vi "Teleop.vi"(10 "Match Info":T1={"Autonomous Elapsed Seconds"=0.0, "TeleOp Elapsed Seconds"=0.0, "Disabled Elapsed Seconds"=0.0, "Visited Autonomous"=FALSE, "Visited TeleOp"=FALSE, "Visited Disabled"=FALSE, "Autonomous Settings"={"Autonomous Style"=enum."Independent", "VI Refnum"=refnum}}, 11 "Call Context":T2) -> ()   [LabVIEW 2011]
doc: "This VI is called for each TeleOp packet received from the DS where the robot is not disabled. It is often used to read from the joysticks and update I/O or to update setpoints for timed control loops. It should complete and return within 20 milliseconds or it may miss DS packets."
uses:
  <vilib>/Rock Robotics/WPI/DriverStation/WPI_DriverStationDerivedRobotMode.ctl
  <vilib>/Rock Robotics/WPI/DriverStation/WPI_DriverStationMatch Info.ctl
  Robot Global Data.vi
  System Set Points and States.vi
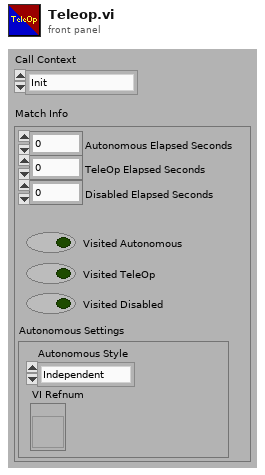
[diagram p1: front panel]
types:
  T1 = typedef "WPI_DriverStationMatch Info.ctl" = cluster{"Autonomous Elapsed Seconds":dbl, "TeleOp Elapsed Seconds":dbl, "Disabled Elapsed Seconds":dbl, "Visited Autonomous":bool, "Visited TeleOp":bool, "Visited Disabled":bool, "Autonomous Settings":cluster{"Autonomous Style":enum16{"Iterative", "Independent"}, "VI Refnum":refnum<vi>}}
  T2 = typedef "WPI_DriverStationDerivedRobotMode.ctl" = enum16{"Init", "Execute", "Stop"}
  T3 = typedef "WPI_JoystickDevRef.ctl" = cluster{"Device":T4}
  T4 = typedef "WPI_JoystickDeviceEnum.ctl" = enum16{"USB 1", "USB 2", "USB 3", "USB 4", "Kinect 1", "Kinect 2"}
  T5 = typedef "WPI_JoystickButtonState.ctl" = cluster{"Button 1":bool, "Button 2":bool, "Button 3":bool, "Button 4":bool, "Button 5":bool, "Button 6":bool, "Button 7":bool, "Button 8":bool, "Button 9":bool, "Button 10":bool, "Button 11":bool, "Button 12":bool}
  T6 = cluster{"axis 1 (x)":dbl, "axis 2 (y)":dbl, "axis 3 (throttle)":dbl, "axis 4":dbl, "axis 5":dbl, "axis 6":dbl}
  T7 = typedef "WPI_DigitalInputDevRef.ctl" = cluster{"DevStatus":errorcluster, "DIO Channel":T8, "Digital Module":T9}
  T8 = typedef "FPGA_DIOChannel.ctl" = enum8{"DIO 1", "DIO 2", "DIO 3", "DIO 4", "DIO 5", "DIO 6", "DIO 7", "DIO 8", "DIO 9", "DIO 10", "DIO 11", "DIO 12", "DIO 13", "DIO 14", "Invalid"}
  T9 = typedef "FPGA_TypedefDigitalModule.ctl" = enum16{"Digital Module 1", "Digital Module 2"}
  T10 = typedef "WPI_RobotDriveDevRef.ctl" = cluster{"DevStatus":errorcluster, "Motors[]":T11[], "Square Inputs":bool, "Max Output":dbl, "Isochronous":bool}
  T11 = typedef "WPI_MotorControlDeviceRef.ctl" = cluster{"DeviceStatus":errorcluster, "Type":enum16{"PWM", "CAN"}, "PWM":cluster{"Digital Module":T9, "PWM Channel":T12, "DeadBand":T13}, "CAN":cluster{"Device Number":u8, "Control Mode":T14, "Semaphore":T15, "Max Vout":dbl}, "Invert":bool, "TransformRef":T16, "InvTransformRef":T16}
  T12 = typedef "FPGA_DIOPWMChannel.ctl" = enum8{"PWM 1", "PWM 2", "PWM 3", "PWM 4", "PWM 5", "PWM 6", "PWM 7", "PWM 8", "PWM 9", "PWM 10", "Invalid"}
  T13 = typedef "WPI_PWMDeadband.ctl" = cluster{"Name":string, "maxPositivePwm":i32, "minPositivePwm":i32, "centerPwm":i32, "maxNegativePwm":i32, "minNegativePwm":i32, "angularRange":u16}
  T14 = typedef "WPI_CANJaguar_ControlMode.ctl" = enum8{"Percent VBus", "Current", "Speed", "Position", "Voltage"}
  T15 = typedef "Semaphore RefNum" = refnum<k1>
  T16 = typedef "WPI_PWMTransform_ConPane.ctl" = refnum<vi>
  T17 = cluster{"Position":cluster{"X":dbl, "Y":dbl}, "Distance (ft)":dbl}[]
  T18 = cluster{"Target Info[0]":cluster{"Position":cluster{"X":dbl, "Y":dbl}, "Distance (ft)":dbl}, "Target Info[1]":cluster{"Position":cluster{"X":dbl, "Y":dbl}, "Distance (ft)":dbl}, "Target Info[2]":cluster{"Position":cluster{"X":dbl, "Y":dbl}, "Distance (ft)":dbl}, "Target Info[3]":cluster{"Position":cluster{"X":dbl, "Y":dbl}, "Distance (ft)":dbl}, "Target Info[4]":cluster{"Position":cluster{"X":dbl, "Y":dbl}, "Distance (ft)":dbl}, "Target Info[5]":cluster{"Position":cluster{"X":dbl, "Y":dbl}, "Distance (ft)":dbl}, "Target Info[6]":cluster{"Position":cluster{"X":dbl, "Y":dbl}, "Distance (ft)":dbl}, "Target Info[7]":cluster{"Position":cluster{"X":dbl, "Y":dbl}, "Distance (ft)":dbl}, "Target Info[8]":cluster{"Position":cluster{"X":dbl, "Y":dbl}, "Distance (ft)":dbl}}
  T19 = typedef "WPI_AnalogChannelDevRef.ctl" = cluster{"DevStatus":errorcluster, "Analog Module":T20, "Analog Channel":T21}
  T20 = typedef "FPGA_TypedefAnalogModule.ctl" = enum16{"Analog Module 1", "Analog Module 2"}
  T21 = typedef "FPGA_AIChannel.ctl" = enum8{"AI 1", "AI 2", "AI 3", "AI 4", "AI 5", "AI 6", "AI 7", "AI 8", "Invalid"}
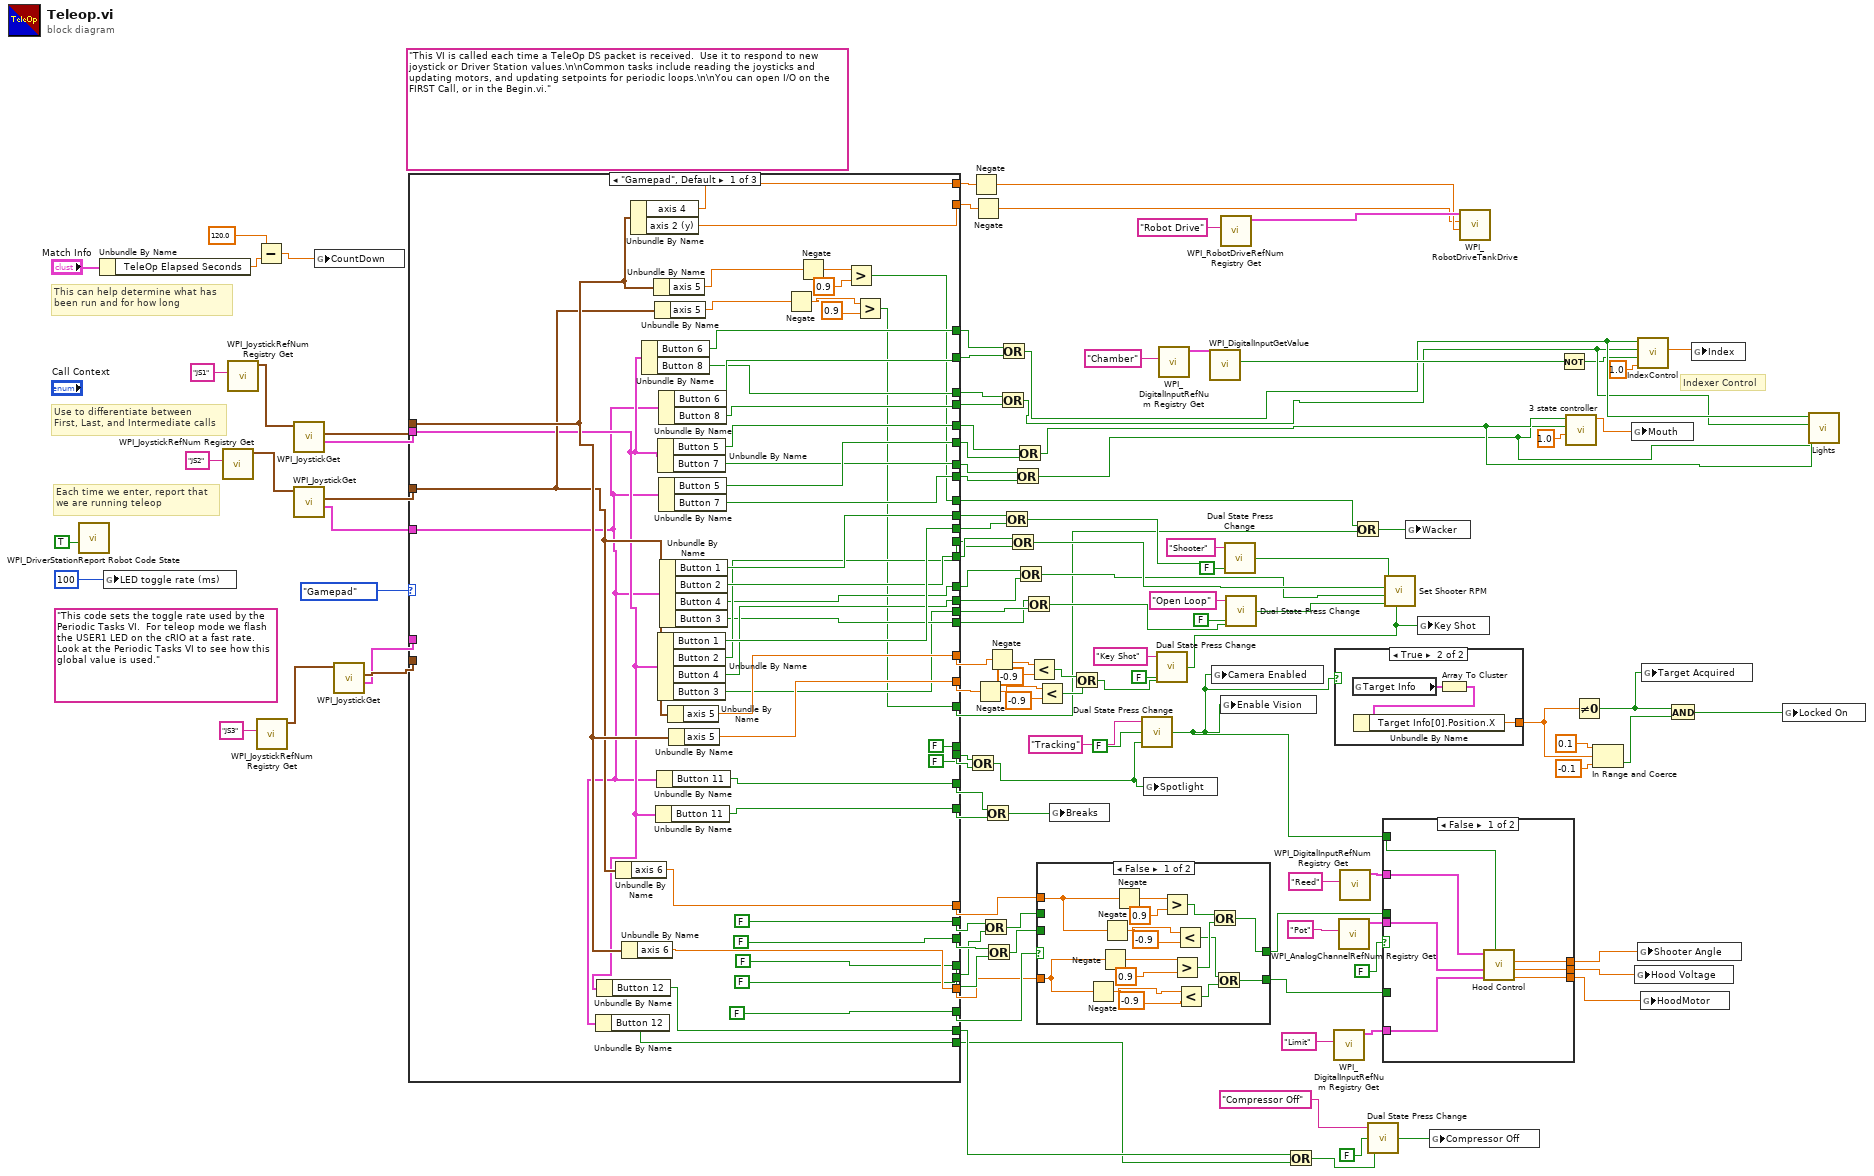
[diagram p0: block diagram]
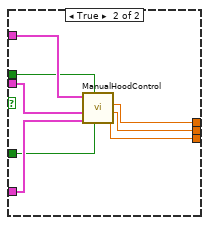
[diagram p2: hidden frame]
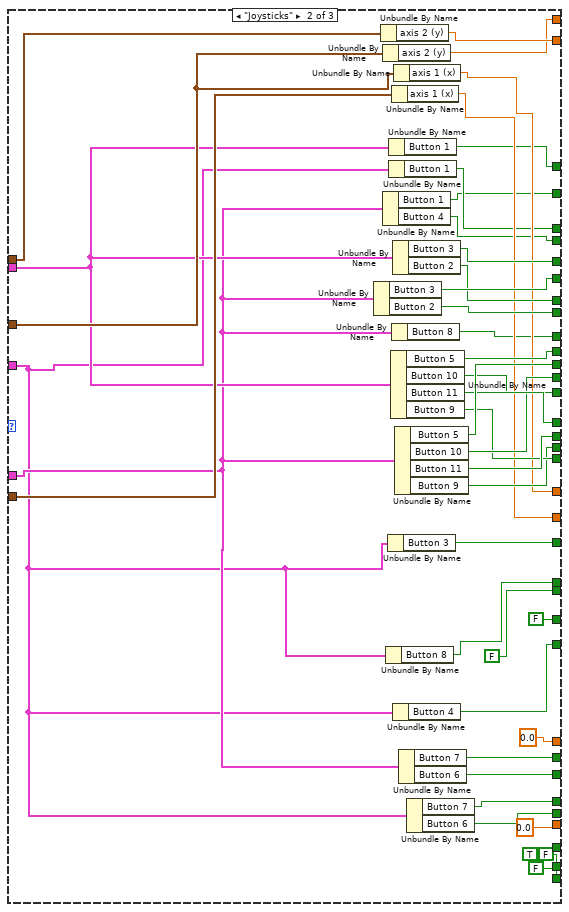
[diagram p4: hidden frame]
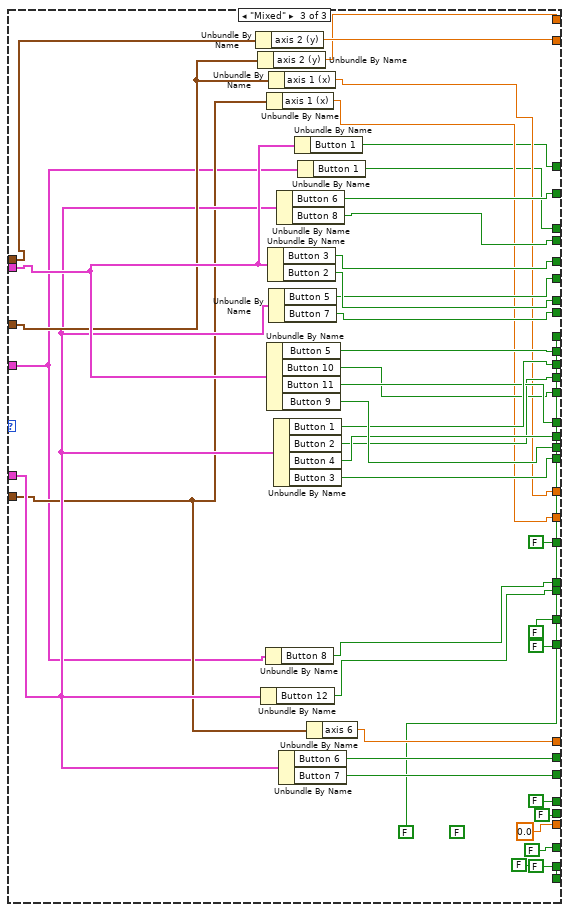
[diagram p5: hidden frame]
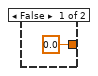
[diagram p6: hidden frame]
diagram:
  (unwired) "This code sets the toggle rate used by the Periodic Tasks VI.  For teleop mode we flash the USER1 LED on the cRIO at a fast rate.  Look at the Periodic Tasks VI to see how this global value is used."
  (unwired) "This VI is called each time a TeleOp DS packet is received.  Use it to respond to new joystick or Driver Station values.\n\nCommon tasks include reading the joysticks and updating motors, and updating setpoints for periodic loops.\n\nYou can open I/O on the FIRST Call, or in the Begin.vi."
  # "Indexer Control"
  # "Each time we enter, report that\nwe are running teleop"
  # "Use to differentiate between\nFirst, Last, and Intermediate calls"
  # "This can help determine what has\nbeen run and for how long"
  n1 = call <vilib>:"WPI_DriverStationReport Robot Code State.vi"("TeleOp"=TRUE ("Autonomous")) -> ()  [unwired: 10 in, 1 out]
  n2 = Unbundle By Name("Match Info") -> ("TeleOp Elapsed Seconds"=w95:dbl)
  n3 = global write "Robot Global Data.vi" "LED toggle rate (ms)"(u32 100 ("LED ms toggle rate")) -> ()
  n4 = call <vilib>:"WPI_JoystickRefNum Registry Get.vi"("refnum name"="JS2") -> ("JoystickDevRef"=w89:T3)  [unwired: 9 in, 1 out]
  n5 = call <vilib>:"WPI_JoystickRefNum Registry Get.vi"("refnum name"="JS1") -> ("JoystickDevRef"=w116:T3)  [unwired: 9 in, 1 out]
  n6 = Subtract(x=120.0, y=w95) -> (x-y=w61:dbl)
  n7 = call <vilib>:"WPI_JoystickRefNum Registry Get.vi"("refnum name"="JS3") -> ("JoystickDevRef"=w57:T3)  [unwired: 9 in, 1 out]
  n8 = call <vilib>:"WPI_JoystickGet.vi"("JoystickDevRef"=w116) -> ("Buttons"=w103:T5, "Axes"=w62:T6)  [unwired: 4 in, 1 out]
  n9 = call <vilib>:"WPI_JoystickGet.vi"("JoystickDevRef"=w89) -> ("Buttons"=w69:T5, "Axes"=w63:T6)  [unwired: 4 in, 1 out]
  n10 = global write "System Set Points and States.vi" "CountDown"(w61) -> ()
  n11 = call <vilib>:"WPI_JoystickGet.vi"("JoystickDevRef"=w57) -> ("Buttons"=w59:T5, "Axes"=w60:T6)  [unwired: 4 in, 1 out]
  n12 = case shown="\"Gamepad\", Default" enum16{"Gamepad", "Mixed", "Joysticks"}."Gamepad" {
    tunnel: [w165 w181 w218] -> w113
    tunnel: [w164 w182 w219] -> w112
    tunnel: w103 -> [w124 w180 w246]
    tunnel: [w163 0.0 ("axis 6") 0.0 ("axis 6")] -> w8
    tunnel: [w162 w199 w238] -> w88
    tunnel: [w161 w200 w237] -> w87
    tunnel: [w160 w197 w233] -> w85
    tunnel: [w159 w196 w234] -> w84
    tunnel: [w158 w195 w235] -> w82
    tunnel: [w157 w198 w236] -> w81
    tunnel: [w139 w193 w239] -> w79
    tunnel: [w156 w194 w240] -> w78
    tunnel: [w155 w176 w227] -> w76
    tunnel: [w154 w179 w216] -> w75
    tunnel: [w153 w178 w215] -> w73
    tunnel: [w152 w175 w228] -> w72
    tunnel: [w151 w192 w229] -> w70
    tunnel: w69 -> [w123 w170 w217]
    tunnel: [w142 w190 w231] -> w41
    tunnel: [w143 w191 w230] -> w42
    tunnel: [w150 w189 w232] -> w67
    tunnel: [FALSE ("Button 8") w201 w241] -> w65
    tunnel: [FALSE ("Button 12") FALSE ("Button 12") w223] -> w64
    tunnel: [w149 0.0 ("axis 6") w220] -> w9
    tunnel: w63 -> [w137 w183 w224]
    tunnel: w62 -> [w138 w205 w247]
    tunnel: w60 -> [_ w206 w221]
    tunnel: w59 -> [_ w174 w222]
    tunnel: [w147 w188 w226] -> w50
    tunnel: [w148 w187 w225] -> w49
    tunnel: [FALSE ("Button 6") w186 w243] -> w26
    tunnel: [FALSE ("Button 7") w185 w242] -> w30
    tunnel: [FALSE TRUE FALSE] -> w48
    tunnel: [w130 w177 FALSE ("Button 1")] -> w32
    tunnel: [w129 w173 FALSE ("Button 3")] -> w33
    tunnel: [FALSE ("Button 7") w172 FALSE ("Button 7")] -> w29
    tunnel: [FALSE ("Button 6") w171 FALSE ("Button 6")] -> w27
    tunnel: [w126 FALSE ("Button 12") FALSE ("Button 4")] -> w20
    tunnel: [w125 w169 FALSE ("Button 4")] -> w19
    tunnel: [w122 FALSE ("Button 11") FALSE ("Button 11")] -> w5
    tunnel: [w121 FALSE ("Button 11") FALSE ("Button 11")] -> w4
    frame "Gamepad", Default {
      n13 = Unbundle By Name(w123) -> ("Button 12"=w121:bool)
      n14 = Unbundle By Name(w124) -> ("Button 12"=w122:bool)
      n15 = Unbundle By Name(w137) -> ("axis 6"=w149:dbl)
      n16 = Unbundle By Name(w138) -> ("axis 6"=w163:dbl)
      n17 = Unbundle By Name(w138) -> ("axis 4"=w165:dbl, "axis 2 (y)"=w164:dbl)
      n18 = Unbundle By Name(w124) -> ("Button 6"=w154:bool, "Button 8"=w153:bool)
      n19 = Unbundle By Name(w138) -> ("axis 5"=w136:dbl)
      n20 = Unbundle By Name(w137) -> ("axis 5"=w135:dbl)
      n21 = Unbundle By Name(w124) -> ("Button 11"=w125:bool)
      n22 = Unbundle By Name(w123) -> ("Button 11"=w126:bool)
      n23 = Unbundle By Name(w124) -> ("Button 5"=w151:bool, "Button 7"=w142:bool)
      n24 = Unbundle By Name(w124) -> ("Button 1"=w161:bool, "Button 2"=w159:bool, "Button 4"=w158:bool, "Button 3"=w139:bool)
      n25 = Unbundle By Name(w123) -> ("Button 6"=w155:bool, "Button 8"=w152:bool)
      n26 = Unbundle By Name(w123) -> ("Button 5"=w143:bool, "Button 7"=w150:bool)
      n27 = Unbundle By Name(w123) -> ("Button 1"=w162:bool, "Button 2"=w160:bool, "Button 4"=w157:bool, "Button 3"=w156:bool)
      n28 = Unbundle By Name(w137) -> ("axis 5"=w148:dbl)
      n29 = Unbundle By Name(w138) -> ("axis 5"=w147:dbl)
      n30 = Negate(x=w135) -> (-x=w132:dbl)
      n31 = Negate(x=w136) -> (-x=w134:dbl)
      n32 = Greater?(x=w134, y=0.9) -> (0:w130:bool)
      n33 = Greater?(x=w132, y=0.9) -> (0:w129:bool)
    }
    frame "Joysticks" {
      n34 = Unbundle By Name(w174) -> ("Button 3"=w191:bool, "Button 2"=w189:bool)
      n35 = Unbundle By Name(w205) -> ("axis 2 (y)"=w182:dbl)
      n36 = Unbundle By Name(w183) -> ("axis 2 (y)"=w181:dbl)
      n37 = Unbundle By Name(w174) -> ("Button 1"=w176:bool, "Button 4"=w175:bool)
      n38 = Unbundle By Name(w170) -> ("Button 8"=w201:bool)
      n39 = Unbundle By Name(w170) -> ("Button 3"=w173:bool)
      n40 = Unbundle By Name(w180) -> ("Button 1"=w179:bool)
      n41 = Unbundle By Name(w170) -> ("Button 1"=w178:bool)
      n42 = Unbundle By Name(w180) -> ("Button 5"=w199:bool, "Button 10"=w197:bool, "Button 11"=w198:bool, "Button 9"=w194:bool)
      n43 = Unbundle By Name(w206) -> ("axis 1 (x)"=w188:dbl)
      n44 = Unbundle By Name(w174) -> ("Button 8"=w177:bool)
      n45 = Unbundle By Name(w180) -> ("Button 3"=w192:bool, "Button 2"=w190:bool)
      n46 = Unbundle By Name(w170) -> ("Button 4"=w169:bool)
      n47 = Unbundle By Name(w183) -> ("axis 1 (x)"=w187:dbl)
      n48 = Unbundle By Name(w174) -> ("Button 5"=w200:bool, "Button 10"=w196:bool, "Button 11"=w195:bool, "Button 9"=w193:bool)
      n49 = Unbundle By Name(w174) -> ("Button 7"=w186:bool, "Button 6"=w185:bool)
      n50 = Unbundle By Name(w170) -> ("Button 7"=w171:bool, "Button 6"=w172:bool)
    }
    frame "Mixed" {
      (unwired) FALSE ("Button 4")
      n51 = Unbundle By Name(w247) -> ("axis 2 (y)"=w219:dbl)
      n52 = Unbundle By Name(w224) -> ("axis 2 (y)"=w218:dbl)
      n53 = Unbundle By Name(w222) -> ("Button 12"=w223:bool)
      n54 = Unbundle By Name(w217) -> ("Button 8"=w241:bool)
      n55 = Unbundle By Name(w221) -> ("axis 1 (x)"=w226:dbl)
      n56 = Unbundle By Name(w246) -> ("Button 5"=w238:bool, "Button 10"=w233:bool, "Button 11"=w236:bool, "Button 9"=w239:bool)
      n57 = Unbundle By Name(w246) -> ("Button 3"=w229:bool, "Button 2"=w231:bool)
      n58 = Unbundle By Name(w224) -> ("axis 1 (x)"=w225:dbl)
      n59 = Unbundle By Name(w222) -> ("Button 5"=w230:bool, "Button 7"=w232:bool)
      n60 = Unbundle By Name(w222) -> ("Button 1"=w237:bool, "Button 2"=w234:bool, "Button 4"=w235:bool, "Button 3"=w240:bool)
      n61 = Unbundle By Name(w222) -> ("Button 6"=w227:bool, "Button 8"=w228:bool)
      n62 = Unbundle By Name(w222) -> ("Button 6"=w243:bool, "Button 7"=w242:bool)
      n63 = Unbundle By Name(w246) -> ("Button 1"=w216:bool)
      n64 = Unbundle By Name(w217) -> ("Button 1"=w215:bool)
      n65 = Unbundle By Name(w221) -> ("axis 6"=w220:dbl)
    }
  }
  n66 = Or(x=w65, y=w64) -> (x .or. y?=w38:bool)
  n67 = Negate(x=w113) -> (-x=w44:dbl)
  n68 = Negate(x=w112) -> (-x=w43:dbl)
  n69 = Negate(x=w50) -> (-x=w53:dbl)
  n70 = Or(x=w26, y=w27) -> (x .or. y?=w28:bool)
  n71 = Or(x=w20, y=w19) -> (x .or. y?=w21:bool)
  n72 = Or(x=w30, y=w29) -> (x .or. y?=w31:bool)
  n73 = Negate(x=w49) -> (-x=w55:dbl)
  n74 = Or(x=w73, y=w72) -> (x .or. y?=w71:bool)
  n75 = Or(x=w75, y=w76) -> (x .or. y?=w74:bool)
  n76 = Or(x=w88, y=w87) -> (x .or. y?=w86:bool)
  n77 = Or(x=w85, y=w84) -> (x .or. y?=w83:bool)
  n78 = Or(x=w41, y=w67) -> (x .or. y?=w66:bool)
  n79 = Or(x=w70, y=w42) -> (x .or. y?=w68:bool)
  n80 = Or(x=w81, y=w82) -> (x .or. y?=w80:bool)
  n81 = Or(x=w78, y=w79) -> (x .or. y?=w77:bool)
  n82 = Less?(x=w55, y=-0.9) -> (x < y?=w52:bool)
  n83 = Less?(x=w53, y=-0.9) -> (x < y?=w51:bool)
  n84 = case shown="False" w48 {
    tunnel: w8 -> [w254 _]
    tunnel: w9 -> [w255 _]
    tunnel: [w251 w264] -> w11
    tunnel: [w248 w265] -> w10
    tunnel: w28 -> [_ w265]
    tunnel: w31 -> [_ w264]
    frame False {
      n85 = Negate(x=w254) -> (-x=w259:dbl)
      n86 = Negate(x=w254) -> (-x=w261:dbl)
      n87 = Negate(x=w255) -> (-x=w256:dbl)
      n88 = Negate(x=w255) -> (-x=w263:dbl)
      n89 = Greater?(x=w263, y=0.9) -> (0:w253:bool)
      n90 = Greater?(x=w261, y=0.9) -> (0:w252:bool)
      n91 = Less?(x=w256, y=-0.9) -> (x < y?=w250:bool)
      n92 = Less?(x=w259, y=-0.9) -> (x < y?=w249:bool)
      n93 = Or(x=w253, y=w252) -> (x .or. y?=w251:bool)
      n94 = Or(x=w250, y=w249) -> (x .or. y?=w248:bool)
    }
    frame True {
    }
  }
  n95 = global write "System Set Points and States.vi" "Breaks"(w21) -> ()
  n96 = Or(x=w52, y=w51) -> (x .or. y?=w45:bool)
  n97 = call "Dual State Press Change.vi"("Enable/Disable"=w38, "Initial"=FALSE, "Value Name"="Tracking") -> ("Enabled"=w93:bool)
  n98 = global write "System Set Points and States.vi" "Spotlight"(w38) -> ()
  n99 = call "Dual State Press Change.vi"("Enable/Disable"=w45, "Initial"=FALSE, "Value Name"="Key Shot") -> ("Enabled"=w18:bool)
  n100 = call <vilib>:"WPI_DigitalInputRefNum Registry Get.vi"("refnum name"="Chamber") -> ("DigitalInputDevRef"=w111:T7)  [unwired: 9 in, 1 out]
  n101 = call <vilib>:"WPI_DigitalInputGetValue.vi"("DigitalInputDevRef"=w111) -> ("Value"=w109:bool)  [unwired: 8 in, 2 out]
  n102 = global write "System Set Points and States.vi" "Camera Enabled"(w93) -> ()
  n103 = call <vilib>:"WPI_RobotDriveRefNum Registry Get.vi"("refnum name"="Robot Drive") -> ("RobotDriveDevRef"=w114:T10)  [unwired: 9 in, 1 out]
  n104 = global write "Robot Global Data.vi" "Enable Vision"(w93) -> ()
  n105 = call "Dual State Press Change.vi"("Enable/Disable"=w86, "Initial"=FALSE, "Value Name"="Shooter") -> ("Enabled"=w39:bool)
  n106 = call "Dual State Press Change.vi"("Enable/Disable"=w77, "Initial"=FALSE, "Value Name"="Open Loop") -> ("Enabled"=w104:bool)
  n107 = Or(x=w5, y=w4) -> (x .or. y?=w2:bool)
  n108 = call <vilib>:"WPI_DigitalInputRefNum Registry Get.vi"("refnum name"="Limit") -> ("DigitalInputDevRef"=w14:T7)  [unwired: 9 in, 1 out]
  n109 = case shown="True" w93 {
    tunnel: [0.0 ("Distance (ft)") w267] -> w96
    frame False {
    }
    frame True {
      n110 = global read "Robot Global Data.vi" "Target Info"() -> (w269:T17)
      n111 = Array To Cluster(array=w269) -> (cluster=w268:T18)
      n112 = Unbundle By Name(w268) -> ("Target Info[0].Position.X"=w267:dbl)
    }
  }
  n113 = call <vilib>:"WPI_AnalogChannelRefNum Registry Get.vi"("refnum name"="Pot") -> ("AIDeviceRef"=w12:T19)  [unwired: 9 in, 1 out]
  n114 = call <vilib>:"WPI_DigitalInputRefNum Registry Get.vi"("refnum name"="Reed") -> ("DigitalInputDevRef"=w15:T7)  [unwired: 9 in, 1 out]
  n115 = Or(x=w32, y=w33) -> (x .or. y?=w25:bool)
  n116 = call "Dual State Press Change.vi"("Enable/Disable"=w2, "Initial"=FALSE, "Value Name"="Compressor Off") -> ("Enabled"=w1:bool)
  n117 = case shown="False" FALSE {
    tunnel: w93 -> [w276 _]
    tunnel: [w275 w279] -> w92
    tunnel: [w274 w278] -> w91
    tunnel: [w273 w277] -> w22
    tunnel: w15 -> [w272 w283]
    tunnel: w14 -> [w271 w284]
    tunnel: w12 -> [w270 w282]
    tunnel: w11 -> [_ w281]
    tunnel: w10 -> [_ w280]
    frame False {
      n118 = call "Hood Control.vi"("Vision"=w276, "Top"=w271, "AIDeviceRef"=w270, "Bottom"=w272) -> ("HoodSpeed"=w273:dbl, "Voltage"=w274:dbl, "Shoter Angle"=w275:dbl)  [unwired: 5 in]
    }
    frame True {
      n119 = call "ManualHoodControl.vi"("Down"=w280, "Up"=w281, "Top"=w284, "AIDeviceRef"=w282, "Bottom"=w283) -> ("Hood Speed"=w277:dbl, "Voltage"=w278:dbl, "Shoter Angle"=w279:dbl)  [unwired: 4 in]
    }
  }
  n120 = call "Set Shooter RPM.vi"("Key Shot"=w18, "Open Loop"=w104, "Increment"=w80, "Decrement"=w83, "Shooter Enabled"=w39) -> ()  [unwired: 7 in]
  n121 = global write "System Set Points and States.vi" "Wacker"(w25) -> ()
  n122 = global write "System Set Points and States.vi" "Key Shot"(w18) -> ()
  n123 = global write "System Set Points and States.vi" "Compressor Off"(w1) -> ()
  n124 = call <vilib>:"WPI_RobotDriveTankDrive.vi"("Right axis value"=w44, "Left axis value"=w43, "RobotDriveDevRef"=w114) -> ()  [unwired: 7 in, 2 out]
  n125 = Not(x=w109) -> (.not. x?=w35:bool)
  n126 = call "3 state controller.vi"("Power"=1.0, "Backward"=w66, "Forward"=w68) -> ("Numeric"=w24:dbl)  [unwired: 8 in]
  n127 = Not Equal To 0?(x=w96) -> (x != 0?=w34:bool)
  n128 = In Range and Coerce(upper limit=0.1, x=w96, lower limit=-0.1) -> (In Range?=w98:bool)  [unwired: 1 out]
  n129 = global write "System Set Points and States.vi" "Mouth"(w24) -> ()
  n130 = global write "System Set Points and States.vi" "Hood Voltage"(w91) -> ()
  n131 = call "IndexControl.vi"("Power"=1.0, "Chamber"=w35, "Back"=w71, "Forward"=w74) -> ("Numeric"=w23:dbl)  [unwired: 7 in]
  n132 = global write "System Set Points and States.vi" "Shooter Angle"(w92) -> ()
  n133 = global write "System Set Points and States.vi" "HoodMotor"(w22) -> ()
  n134 = global write "System Set Points and States.vi" "Target Acquired"(w34) -> ()
  n135 = And(x=w34, y=w98) -> (x .and. y?=w97:bool)
  n136 = global write "System Set Points and States.vi" "Index"(w23) -> ()
  n137 = global write "System Set Points and States.vi" "Locked On"(w97) -> ()
  n138 = call "Lights.vi"("Input4"=w68, "Input3"=w66, "Input2"=w71, "Input1"=w74) -> ()  [unwired: 8 in]
